vi "arrayheader.vi"(10 "Numeric":u32 format="%.0x") -> (2 "header":u8[](array[numeric]) format="%.0x")   [LabVIEW 2016, in "MsgPack.lvlib"]
uses:
  MsgPack.lvlib
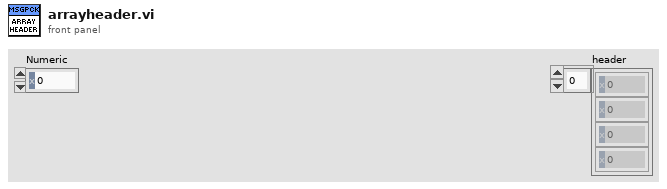
[diagram p1: front panel]
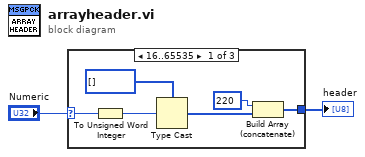
[diagram p0: block diagram]
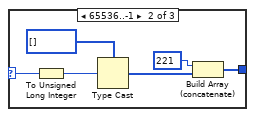
[diagram p2: hidden frame]
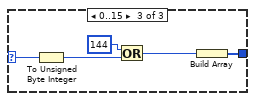
[diagram p3: hidden frame]
diagram:
  n1 = case shown="16..65535" "Numeric" {
    selector: "Numeric" -> [w8 w9 w17]
    tunnel: [w3 w11 w15] -> w2
    frame 16..65535 {
      n2 = To Unsigned Word Integer(number=w8) -> (unsigned 16bit integer=w6:u16)
      n3 = Type Cast(type=u8[] [], x=w6) -> (*(type *) &x=w4:u8[])
      n4 = Build Array (concatenate)(u8 220 ("x"), w4) -> (w3:u8[])
    }
    frame 65536..-1 {
      n5 = To Unsigned Long Integer(number=w9) -> (unsigned 32bit integer=w10:u32)
      n6 = Type Cast(type=u8[] [], x=w10) -> (*(type *) &x=w14:u8[])
      n7 = Build Array (concatenate)(u8 221 ("x"), w14) -> (w11:u8[])
    }
    frame 0..15 {
      n8 = To Unsigned Byte Integer(number=w17) -> (unsigned 8bit integer=w19:u8)
      n9 = Or(x=u8 144, y=w19) -> (x .or. y?=w16:u8)
      n10 = Build Array(w16) -> (w15:u8[])
    }
  }
  "header" <- w2
